vi "json Parse U32 Array - array path.vi"(8 "error in (no error)":errorcluster, 9 "default":u32[](array[numeric]), 10 "path":string[](array[string]), 11 "JSON Document in":refnum<class "JSON Document.lvclass">) -> (0 "error out":errorcluster, 1 "found?":bool, 2 "value":u32[](array[numeric]), 3 "JSON Document out":refnum<class "JSON Document.lvclass">, 4 "size":i32)   [LabVIEW 2015, in "JSON Document.lvclass"]
uses:
  JSON Document.lvclass
  json Parse U32 Array - string path.vi
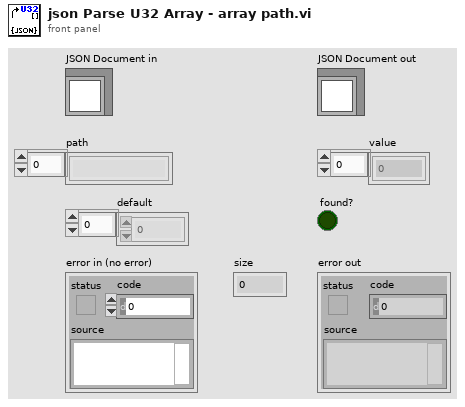
[diagram p1: front panel]
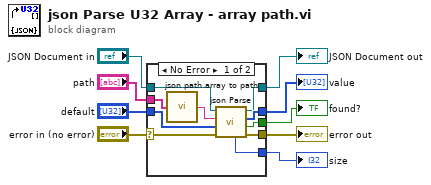
[diagram p0: block diagram]
diagram:
  n1 = case shown="No Error" "error in (no error)" {
    selector: "error in (no error)" -> [w11 w22]
    tunnel: [w10 w22] -> w8
    tunnel: [w15 w21] -> w6
    tunnel: "JSON Document in" -> [w14 w21]
    tunnel: "default" -> [w19 w20]
    tunnel: "path" -> [w13 _]
    tunnel: [w18 w20] -> w3
    tunnel: [w16 _] -> w2
    tunnel: [w17 _] -> w1
    frame No Error {
      n2 = call "json path array to path.vi"("path"=w13) -> ("String"=w12:string)
      n3 = call-poly "json Parse.vi"("error in (no error)"=w11, "default"=w19, "path"=w12, "JSON Document in"=w14) -> ("error out"=w10:errorcluster, "found?"=w16:bool, "value"=w18:u32[], "JSON Document out"=w15:refnum<class "JSON Document.lvclass">, "size"=w17:i32)  [unwired: 3 in]
    }
    frame Error {
    }
  }
  "error out" <- w8
  "JSON Document out" <- w6
  "value" <- w3
  "found?" <- w2
  "size" <- w1
